vi "Configure Trigger (Width).vi"(0 "VISA resource name":refnum<visa-resource-name>, 1 "Width Condition (0: Outside)":i32(ring) items=["Outside", "Within"], 5 "Trigger Source (1: Channel1)":i32(ring)=1 items=["Channel1"=1, "Channel2"=2, "Channel3"=3, "Channel4"=4, "DIG0"=20, "DIG1"=21, "DIG2"=22, "DIG3"=23, "DIG4"=24, "DIG5"=25, "DIG6"=26, "DIG7"=27, "DIG8"=28, "DIG9"=29, "DIG10"=30, "DIG11"=31, "DIG12"=32, "DIG13"=33, "DIG14"=34, "DIG15"=35], 7 "Trigger Point (0:End of Pulse)":i32(ring) items=["End of Pulse", "Timeout"], 9 "Trigger Polarity (0: Negative)":i32(ring) items=["Negative", "Positive"], 11 "error in (no error)":errorcluster, 12 "Width (1E-9 s)":dbl=1e-09) -> (4 "VISA resource name out":refnum<visa-resource-name>, 15 "error out":errorcluster)   [LabVIEW 2020, in "Agilent 90000 Series.lvlib"]
doc: "Configures pulse width trigger parameters."
uses:
  Agilent 90000 Series.lvlib
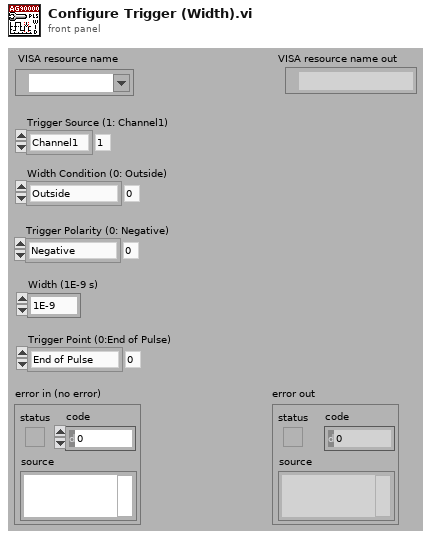
[diagram p1: front panel]
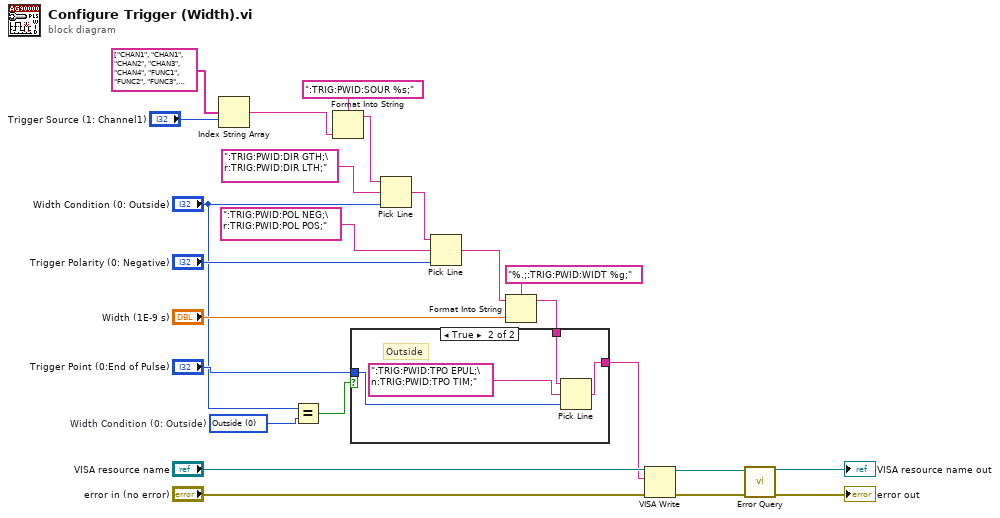
[diagram p0: block diagram]
diagram:
  w5 = 0 items=["Outside", "Within"]  # Width Condition (0: Outside)
  n1 = Index String Array(1:"Trigger Source (1: Channel1)", 2:string[] ["CHAN1", "CHAN1", "CHAN2", "CHAN3", "CHAN4", "FUNC1", "FUNC2", "FUNC3", "FUNC4", "WMEM1", "WMEM2", "WMEM3", "WMEM4", "AUX", "LINE", "", "", "", "", "", "DIG0", "DIG1", "DIG2", "DIG3", "DIG4", "DIG5", "DIG6", "DIG7", "DIG8", "DIG9", "DIG10", "DIG11", "DIG12", "DIG13", "DIG14", "DIG15", "", ""]) -> (0:w11:string)  [unwired: 1 out]
  n2 = Equal?(x="Width Condition (0: Outside)", y=w5) -> (x = y?=w3:bool)
  n3 = Format Into String(format string=":TRIG:PWID:SOUR %s;", w11) -> (resulting string=w10:string)  [unwired: 2 in, 1 out]
  n4 = Pick Line(string ("")=w10, multi-line string=":TRIG:PWID:DIR GTH;\r:TRIG:PWID:DIR LTH;", line index="Width Condition (0: Outside)") -> (output string=w23:string)
  n5 = Pick Line(string ("")=w23, multi-line string=":TRIG:PWID:POL NEG;\r:TRIG:PWID:POL POS;", line index="Trigger Polarity (0: Negative)") -> (output string=w20:string)
  n6 = Format Into String(format string="%.;:TRIG:PWID:WIDT %g;", initial string=w20, "Width (1E-9 s)") -> (resulting string=w7:string)  [unwired: 1 in, 1 out]
  n7 = case shown="True" w3 {
    tunnel: "Trigger Point (0:End of Pulse)" -> [_ w28]
    tunnel: w7 -> [w25 w27]
    tunnel: [w25 w26] -> w6
    frame False {
      # "Within"
    }
    frame True {
      # "Outside"
      n8 = Pick Line(string ("")=w27, multi-line string=":TRIG:PWID:TPO EPUL;\n:TRIG:PWID:TPO TIM;", line index=w28) -> (output string=w26:string)
    }
  }
  n9 = VISA Write(VISA resource name="VISA resource name", write buffer=w6, error in (no error)="error in (no error)") -> (VISA resource name out=w15:refnum<visa-resource-name>, error out=w14:errorcluster)  [unwired: 1 out]
  n10 = call "Error Query.vi"("error in (no error)"=w14, "VISA resource name"=w15) -> ("error out"=→"error out":errorcluster, "VISA resource name out"=→"VISA resource name out":refnum<visa-resource-name>)  [unwired: 8 out]
